vi "SetGearIntakeSpeed.vi"(10 "Gear Intake Speed":dbl) -> ()   [LabVIEW 2016, in "Gear Intake.lvclass"]
uses:
  Gear Intake.lvclass
  Gear Intake.lvclass/Gear Intake.ctl
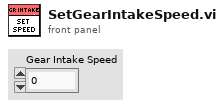
[diagram p1: front panel]
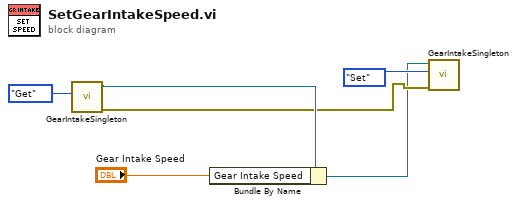
[diagram p0: block diagram]
diagram:
  n1 = call "GearIntakeSingleton.vi"("Get/Set"=enum16{"Get", "Set"}."Get") -> ("error out"=w2:errorcluster, "Gear Intake.lvclass"=w3:refnum<class "Gear Intake.lvclass">)  [unwired: 9 in]
  n2 = Bundle By Name(cluster=w3, "Gear Intake Speed"="Gear Intake Speed") -> (w1:refnum<class "Gear Intake.lvclass">)
  n3 = call "GearIntakeSingleton.vi"("error in (no error)"=w2, "Get/Set"=enum16{"Get", "Set"}."Set", "Gear Intake.lvclass"=w1) -> ()  [unwired: 7 in, 2 out]
